vi "LEBITVacuum.SortAddr.vi"(6 "AMArray in":string[][](array[string])) -> (1 "AMArray out":string[][](array[string]), 2 "MKS Address Array":i32[](array[numeric]))   [LabVIEW 2014, in "LEBITVacuum.lvlib"]
uses:
  LEBITVacuum.lvlib
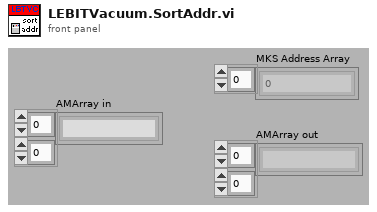
[diagram p1: front panel]
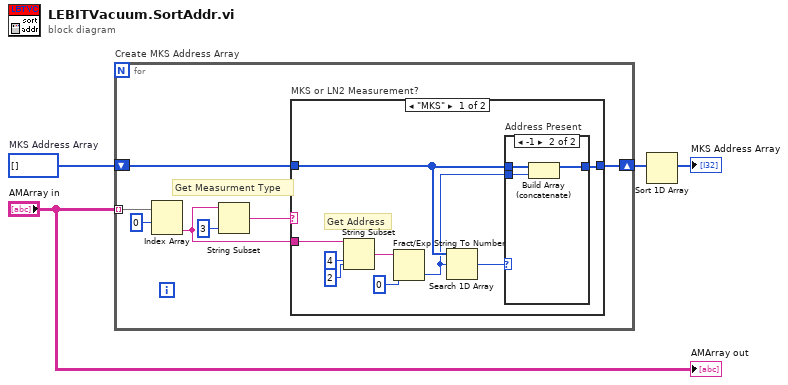
[diagram p0: block diagram]
diagram:
  w2 = i32[] []  # MKS Address Array
  n1 = for "Create MKS Address Array" {
    tunnel: "AMArray in" -> [w11] mode=indexing
    shift-right: [w5] -> w1
    shift-left: w2 -> [w6]
    # "Get Measurment Type"
    n2 = Index Array(array=w11, index #1=0 ("index")) -> (element #2=w7:string)  [unwired: 1 in, 1 out]
    n3 = String Subset(string=w7, length (rest)=3 ("length (rest)")) -> (substring=w8:string)  [unwired: 1 in]
    n4 = case "MKS or LN2 Measurement?" shown="\"MKS\"" w8 {
      tunnel: w6 -> [w14 w25]
      tunnel: w7 -> [w18 _]
      tunnel: [w15 w25] -> w5
      frame "MKS" {
        # "Get Address"
        n5 = String Subset(string=w18, offset (0)=4, length (rest)=2 ("length (rest)")) -> (substring=w17:string)
        n6 = Fract/Exp String To Number(string=w17, default (0 dbl)=0 ("default (0 DBL)")) -> (number=w13:i32)  [unwired: 2 in, 1 out]
        n7 = Search 1D Array(1D array=w14, element=w13) -> (index of element=w16:i32)  [unwired: 1 in]
        n8 = case "Address Present" shown="-1" w16 {
          tunnel: [w21 w24] -> w15
          tunnel: w14 -> [w21 w23]
          tunnel: w13 -> [_ w22]
          frame 0, Default {
          }
          frame -1 {
            n9 = Build Array (concatenate)(w23, w22) -> (w24:i32[])
          }
        }
      }
      frame "LN2", Default {
      }
    }
  }
  n10 = Sort 1D Array(array=w1) -> (sorted array=→"MKS Address Array":i32[])
  "AMArray out" <- "AMArray in"
